vi "AtSpectrograph_ackCommand_changeDisperser.vi"(8 "error in (no error)":errorcluster, 11 "ackcmd_Ctl":T1={"cmdSeqNum"=0, "ack"=0, "error"=0, "result"="                                                                                                                                                                                                                                                                "}) -> (0 "error out":errorcluster, 2 "function return":i32, 3 "ackcmd_Ctl out":T1={"cmdSeqNum"=0, "ack"=0, "error"=0, "result"="                                                                                                                                                                                                                                                                "})   [LabVIEW 2016, in "SALLV_AtSpectrograph.lvlib"]
doc: "int AtSpectrograph_shm_ackCommand_changeDisperserLV(AtSpectrograph_ackcmdLV *ackcmd_Ctl);"
uses:
  SALLV_AtSpectrograph.lvlib
  DataTypes/ackcmd.ctl
  SALLV_AtSpectrograph.so
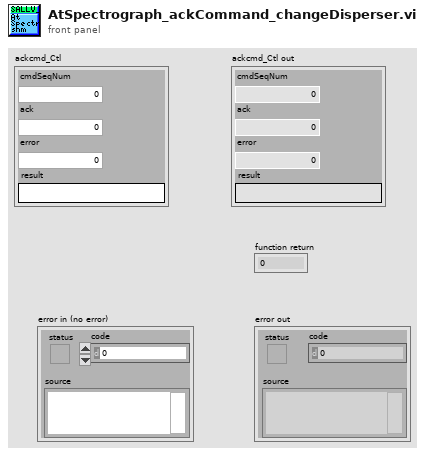
[diagram p1: front panel]
types:
  T1 = typedef "SALLV_AtSpectrograph.lvlib/ackcmd.ctl" = cluster{"cmdSeqNum":i32, "ack":i32, "error":i32, "result":string}
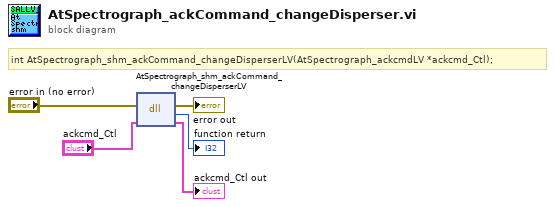
[diagram p0: block diagram]
diagram:
  # "int AtSpectrograph_shm_ackCommand_changeDisperserLV(AtSpectrograph_ackcmdLV *ackcmd_Ctl);"
  n1 = dll-call lib="home/harini/TCS/SALLV_AtSpectrograph/SALLV_AtSpectrograph.*" fn="AtSpectrograph_shm_ackCommand_changeDisperserLV"(error in="error in (no error)", "ackcmd_Ctl"="ackcmd_Ctl") -> (error out=→"error out":errorcluster, →"function return":i32, "ackcmd_Ctl"=→"ackcmd_Ctl out":T1)  [unwired: 2 in, 1 out]
